vi "VisualizeNHRRGS.vi"() -> ()   [LabVIEW 2018, in "Visualization.lvlib" / "VisualizeAcPwr.lvclass"]
uses:
  VisualizeAcPwr.lvclass
  <vilib>/event_ctls.llb/usereventprio.ctl
  VisualizeBase/VisualizeBase_class/Requests/clUserEventType.ctl
  <vilib>/Utility/error.llb/Error Cluster From Error Code.vi
  <vilib>/ErrorRing/Error Ring.xnode
  VisualizeBase/VisualizeBase_class/VisualizeBase.lvclass
  <userlib>/NIST/NISTErrorLib/NISTErrorLib.lvlib
  AcPwr/AcPwrModule/AcPwrModule.lvlib
panel:
  out "Status Byte Register":T1(array[cluster])
  out "Incorrect DataType?":bool
  in  "PluginName":string="AcPwr.NHRRGS0"
  in  "PlotYAxis":u32[](array[numeric])=[0, 1, 0] max=1
  out "NHRRGS":waveform(dbl)[](graph)
  out "ErrorArray":errorcluster[](array[cluster])
  in  "QueuName":string="NHRRGSVQ"
  in  "btnStop":bool
  in  "btnReset":bool
  in  "btnClear":bool
  # "0=Left Axis and 1=Right Axis"
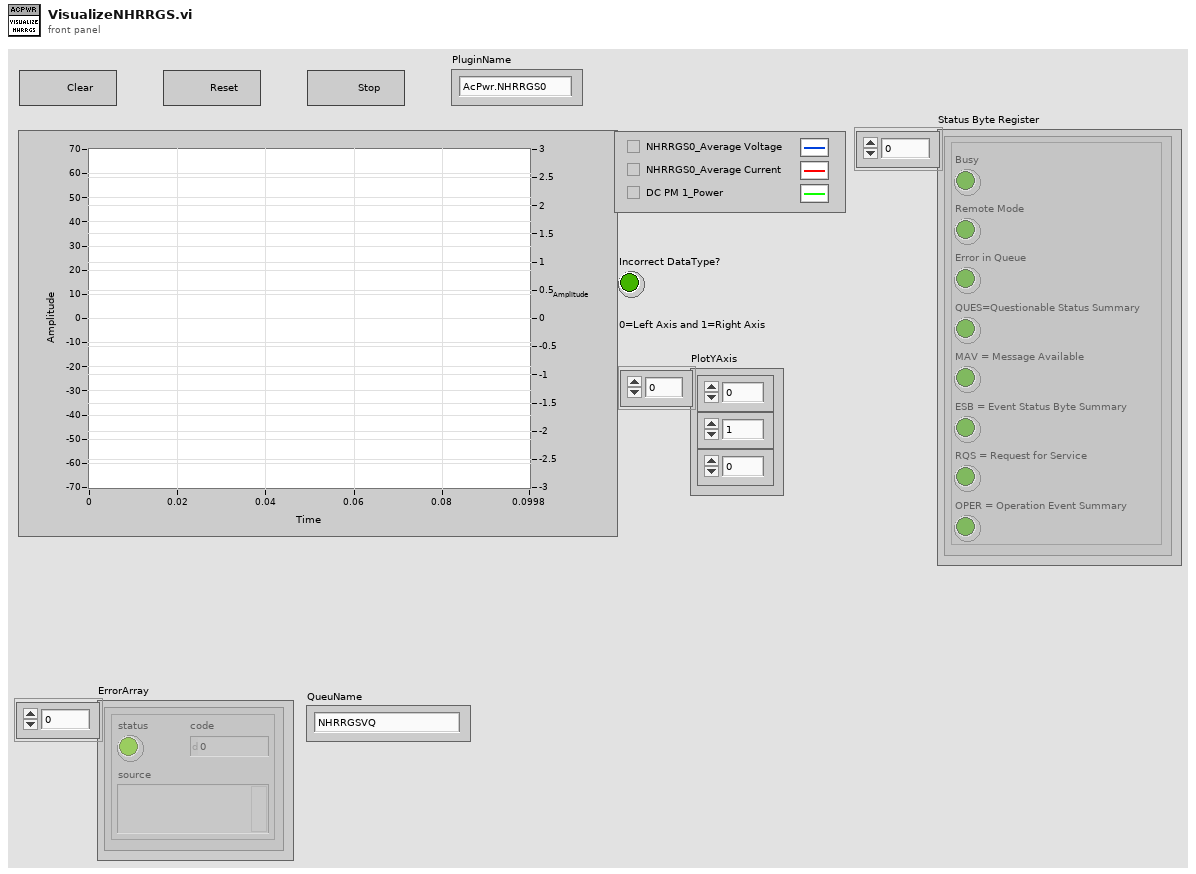
[diagram p1: front panel]
types:
  T1 = cluster{"Busy":bool, "Remote Mode":bool, "Error in Queue":bool, "QUES=Questionable Status Summary":bool, "MAV = Message Available":bool, "ESB = Event Status Byte Summary":bool, "RQS = Request for Service":bool, "OPER = Operation Event Summary":bool}[]
  T2 = typedef "Visualization.lvlib/VisualizeBase.lvclass/clRequestEvents.ctl" = cluster{"StopRequest":refnum<user-event>, "ResetRequest":refnum<user-event>}
  T3 = typedef "AcPwrModule.lvlib/clBroadcastEvents.ctl" = cluster{"DidInit":refnum<user-event>, "StatusUpdate":refnum<user-event>, "ErrorReport":refnum<user-event>, "DidStop":refnum<user-event>, "PathToINI":refnum<user-event>, "Measurements":refnum<user-event>, "LoadConfigFile":refnum<user-event>, "GetSettings":refnum<user-event>, "SetSettings":refnum<user-event>, "GetType&ID":refnum<user-event>, "GotSettings":refnum<user-event>}
  T4 = typedef "Visualization.lvlib/VisualizeBase.lvclass/clUserEventType.ctl" = cluster{"BusIndex":i8, "Data":variant}
  T5 = typedef "usereventprio.ctl" = enum32{"high priority", "normal priority"}
  T6 = cluster{"Busy":bool, "Remote Mode":bool, "Error in Queue":bool, "QUES = Questionable Status Summary":bool, "MAV = Message Available":bool, "ESB = Event Status Byte Summary":bool, "RQS = Request for Service":bool, "OPER = Operation Event Summary":bool}[]
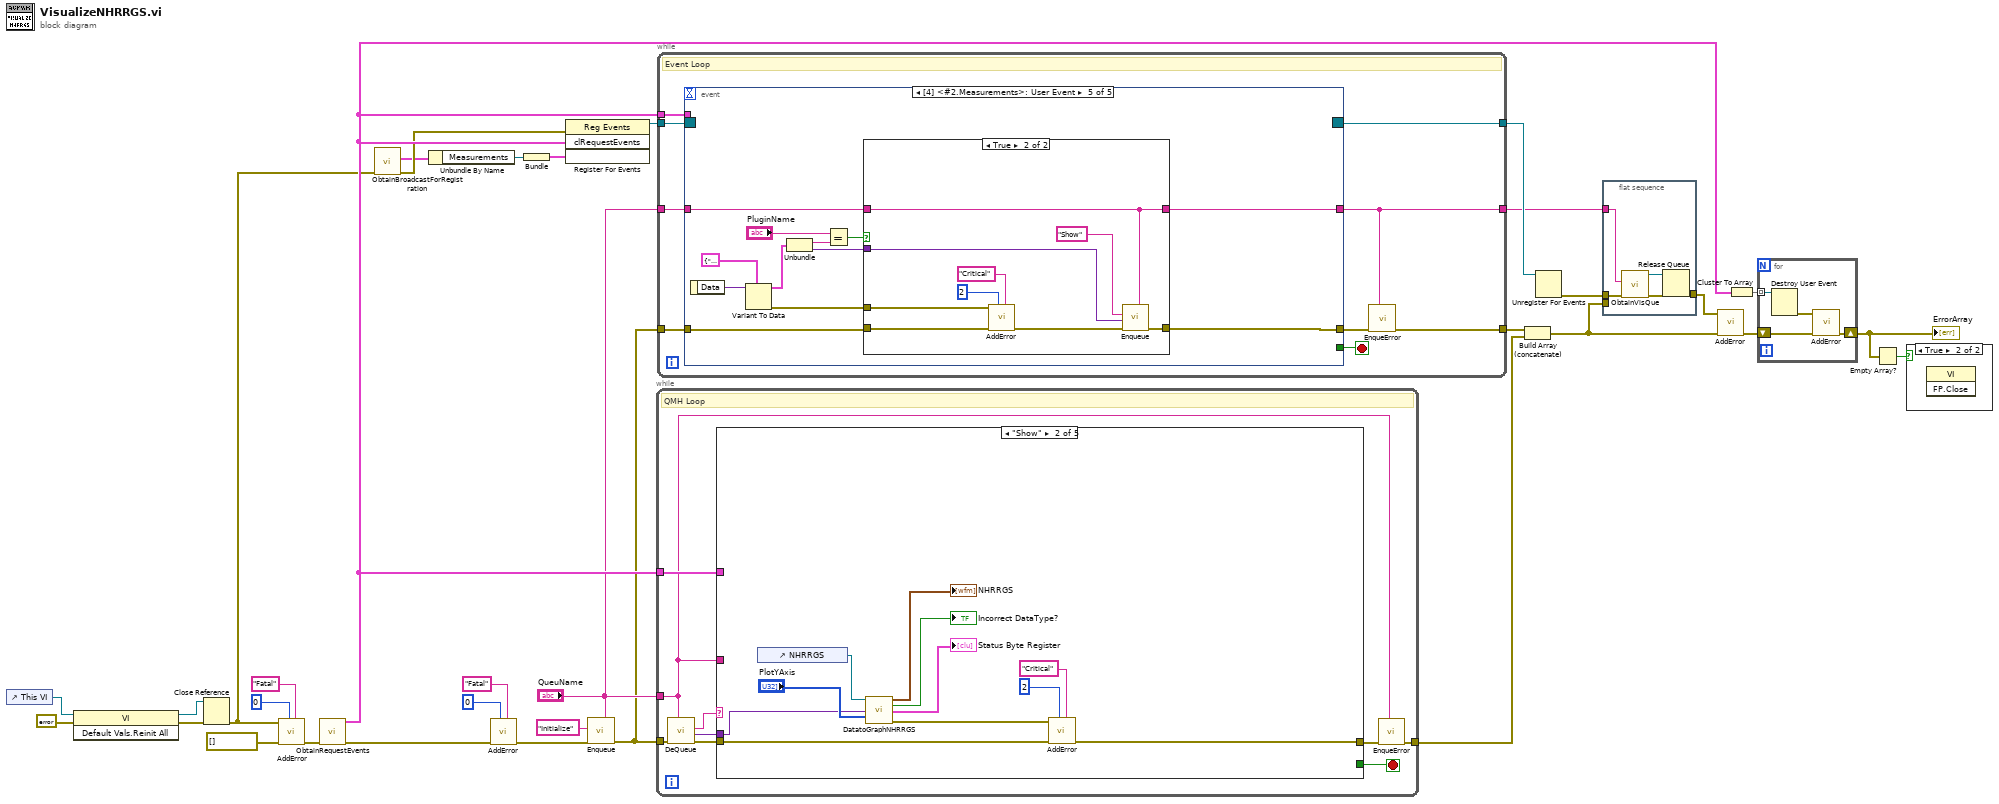
[diagram p0: block diagram]
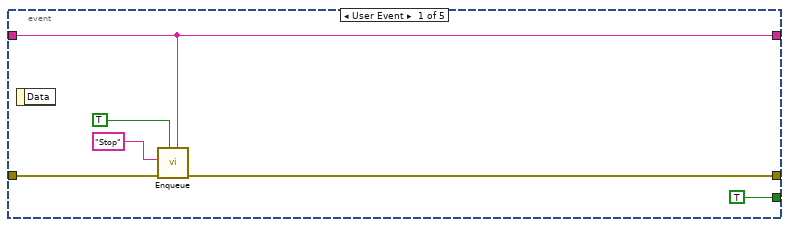
[diagram p2: hidden frame]
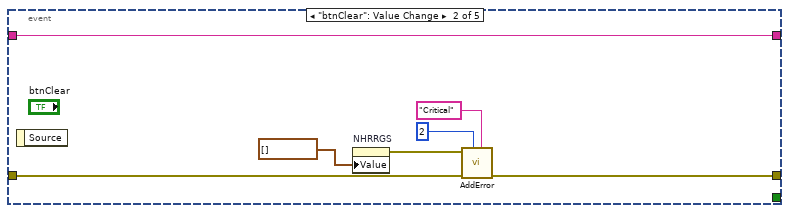
[diagram p3: hidden frame]
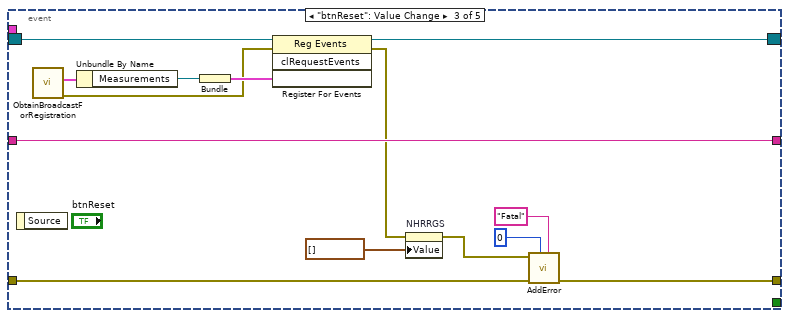
[diagram p4: hidden frame]
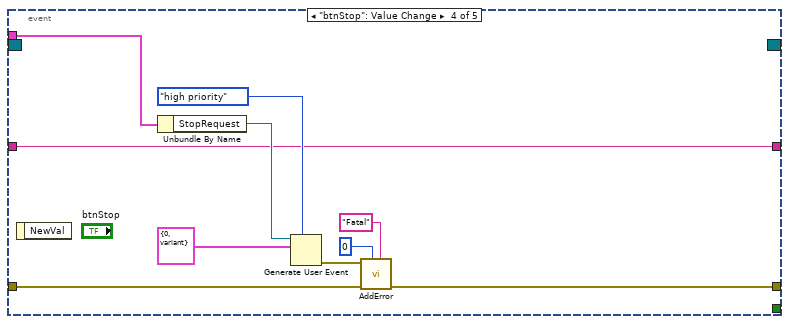
[diagram p5: hidden frame]
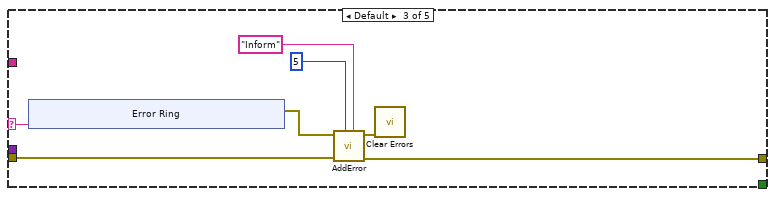
[diagram p8: hidden frame]
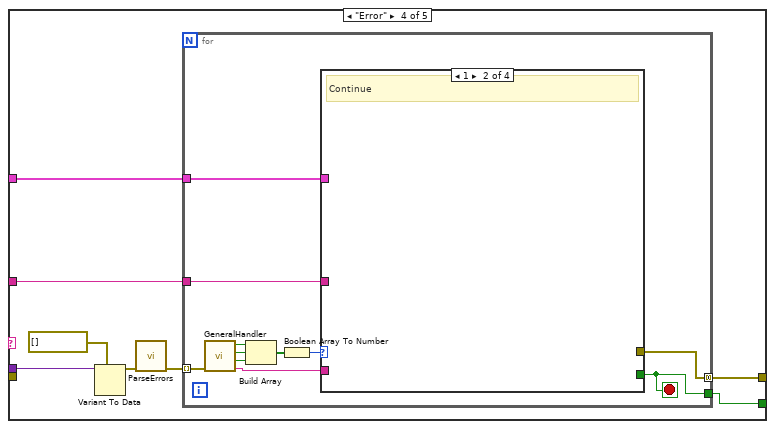
[diagram p9: hidden frame]
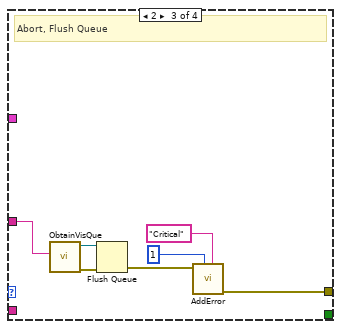
[diagram p11: hidden frame]
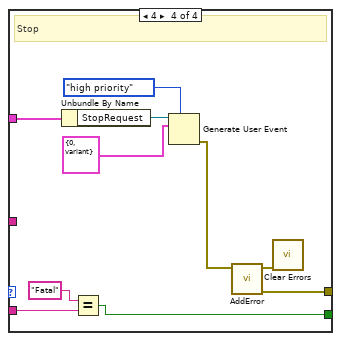
[diagram p12: hidden frame]
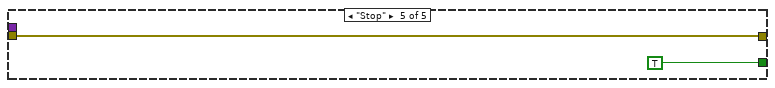
[diagram p13: hidden frame]
diagram:
  n1 = control-ref of="This VI"() -> (w19:refnum<vi>)
  n2 = invoke class="VI" method="Default Vals.Reinit All"(reference=w19, error in=errorcluster {"status"=FALSE, "code"=0, "source"=""} ("error in (no error)")) -> (reference out=w16:refnum<vi>, error out=w17:errorcluster)  [unwired: 1 in, 1 out]
  n3 = Close Reference(reference=w16, error in (no error)=w17) -> (error out=w14:errorcluster)
  n4 = call <userlib>:"AddError.vi"("Severity"="Fatal" ("String"), "Priority"=u8 0, "ErrorArray"=errorcluster[] [], "error in (no error)"=w14) -> ("ErrorArray"=w31:errorcluster[])  [unwired: 6 in, 1 out]
  n5 = call "ObtainRequestEvents.vi"("Error"=w31) -> ("Error"=w4:errorcluster[], "clRequestEvents"=w23:T2)  [unwired: 9 in]
  n6 = call "ObtainBroadcastForRegistration.vi"("error in (no error)"=w14) -> ("error out"=w13:errorcluster, "clBroadcastEvents"=w12:T3)  [unwired: 9 in]
  n7 = Unbundle By Name(w12) -> ("Measurements"=w21:refnum<user-event>)
  n8 = call <userlib>:"AddError.vi"("Severity"="Fatal" ("String"), "Priority"=u8 0, "ErrorArray"=w4) -> ("ErrorArray"=w3:errorcluster[])  [unwired: 7 in, 1 out]
  n9 = Bundle("Measurements"=w21) -> (w20:cluster{"Measurements":refnum<user-event>})  [unwired: 1 in]
  n10 = register-events(error in=w13, w23, w20) -> (reference out=w32:refnum<event-registration>)  [unwired: 1 in, 1 out]
  n11 = call "Enqueue.vi"("QueName"="QueuName", "Error"=w3, "Message"="Initialize") -> ("Error"=w2:errorcluster[])  [unwired: 8 in]
  n12 = while {
    tunnel: w2 -> [w42]
    tunnel: [w36] -> w27
    tunnel: "QueuName" -> [w34]
    tunnel: w23 -> [w35]
    stop <- w37 stop-if-true
    # "QMH Loop"
    n13 = call "DeQueue.vi"("QueName"=w34, "Error"=w42) -> ("Error"=w39:errorcluster[], "Data"=w40:variant, "Message"=w41:string)  [unwired: 7 in]
    n14 = case shown="\"Show\"" w41 {
      selector: w41 -> [_ _ w61 _ _]
      tunnel: w40 -> [_ w45 _ w76 _]
      tunnel: w39 -> [w43 w51 w59 _ w105]
      tunnel: [w43 w54 w58 w72 w105] -> w38
      tunnel: [_ _ _ w71 TRUE] -> w37
      tunnel: w35 -> [_ _ _ w70 _]
      tunnel: w34 -> [_ _ _ w69 _]
      frame "Initialize" {
      }
      frame "Show" {
        n15 = control-ref of="NHRRGS"() -> (w50:refnum<vi>)
        n16 = call "DatatoGraphNHRRGS.vi"("NHRRGS"=w50, "Data"=w45, "PlotYAxis"="PlotYAxis") -> ("WaveformArray"=→"NHRRGS":waveform(dbl)[], "Incorrect DataType?"=→"Incorrect DataType?":bool, "Status Byte Register"=→"Status Byte Register":T6, "error out"=w47:errorcluster)  [unwired: 9 in]
        n17 = call <userlib>:"AddError.vi"("Severity"="Critical" ("String"), "Priority"=u8 2, "ErrorArray"=w51, "error in (no error)"=w47) -> ("ErrorArray"=w54:errorcluster[])  [unwired: 6 in, 1 out]
      }
      frame Default {
        n18 = xnode "Error Ring"("parameter 0"=w61) -> ("error out"=w60:errorcluster)
        n19 = call <userlib>:"AddError.vi"("Severity"="Inform" ("String"), "Priority"=u8 5, "ErrorArray"=w59, "error in (no error)"=w60) -> ("ErrorArray"=w58:errorcluster[], "error out"=w57:errorcluster)  [unwired: 6 in]
        n20 = call <vilib>:"Clear Errors.vi"("error in (no error)"=w57) -> ()  [unwired: 5 in, 2 out]
      }
      frame "Error" {
        n21 = Variant To Data(type=errorcluster[] [], Variant=w76) -> (data=w74:errorcluster[])  [unwired: 1 in, 1 out]
        n22 = call <userlib>:"ParseErrors.vi"("ErrorArray"=w74) -> ("ErrorArray"=w73:errorcluster[])  [unwired: 8 in, 2 out]
        n23 = for {
          tunnel: w73 -> [w87] mode=indexing
          tunnel: [w81] -> w72 mode=concatenating
          tunnel: [w79] -> w71
          tunnel: w70 -> [w78]
          tunnel: w69 -> [w77]
          stop <- w79 stop-if-true
          n24 = call <userlib>:"GeneralHandler.vi"("error in (no error)"=w87) -> ("Severity"=w80:string, "Stop"=w84:bool, "Abort"=w85:bool, "Continue"=w86:bool)  [unwired: 7 in]
          n25 = Build Array(w86, w85, w84) -> (w83:bool[])
          n26 = Boolean Array To Number(Boolean array=w83) -> (number=w82:u32)
          n27 = case shown="1" w82 {
            tunnel: [_ _ w92 w103] -> w81
            tunnel: w80 -> [_ _ _ w98]
            tunnel: [_ _ _ w96] -> w79
            tunnel: w78 -> [_ _ _ w95]
            tunnel: w77 -> [_ _ w88 _]
            frame 0, Default {
              # "No Dialog"
            }
            frame 1 {
              # "Continue"
            }
            frame 2 {
              # "Abort, Flush Queue"
              n28 = call "ObtainVisQue.vi"("QueName"=w88) -> ("error out"=w94:errorcluster, "queue out"=w93:refnum<queue>)  [unwired: 9 in]
              n29 = Flush Queue(queue=w93, error in (no error)=w94) -> (error out=w91:errorcluster)  [unwired: 2 out]
              n30 = call <userlib>:"AddError.vi"("Severity"="Critical" ("String"), "Priority"=u8 1, "error in (no error)"=w91) -> ("ErrorArray"=w92:errorcluster[])  [unwired: 7 in, 1 out]
            }
            frame 4 {
              # "Stop"
              n31 = Unbundle By Name(w95) -> ("StopRequest"=w104:refnum<user-event>)
              n32 = Equal?(x="Fatal", y=w98) -> (x = y?=w96:bool)
              n33 = Generate User Event(priority (normal)=usereventprio."high priority", user event=w104, event data cluster=T4 {"BusIndex"=0, "Data"=variant} ("event data")) -> (error out=w102:errorcluster)  [unwired: 1 in, 1 out]
              n34 = call <userlib>:"AddError.vi"("error in (no error)"=w102) -> ("ErrorArray"=w103:errorcluster[], "error out"=w99:errorcluster)  [unwired: 9 in]
              n35 = call <vilib>:"Clear Errors.vi"("error in (no error)"=w99) -> ()  [unwired: 5 in, 2 out]
            }
          }
        }
      }
      frame "Stop" {
      }
    }
    n36 = call "EnqueError.vi"("QueName"=w34, "Error"=w38) -> ("Error"=w36:errorcluster[])  [unwired: 9 in]
  }
  n37 = while {
    tunnel: w32 -> [w115]
    tunnel: [w112] -> w28
    tunnel: [w111] -> w30
    tunnel: w23 -> [w110]
    tunnel: w2 -> [w109]
    tunnel: "QueuName" -> [w108]
    tunnel: [w107] -> w10
    stop <- w114 stop-if-true
    # "Event Loop"
    n38 = event shown="[4] <#2.Measurements>: User Event" {
      selector: w115 -> [_ _ w142 _ _]
      dyn-events: [_ _ w141 _ _] -> w111
      timeout: _ -> [_ _ _ _ _]
      tunnel: [TRUE _ _ _ _] -> w114
      tunnel: [w120 w125 w135 w150 w164] -> w113
      tunnel: w110 -> [_ _ _ w145 _]
      tunnel: w109 -> [w117 w124 w134 w143 w154]
      tunnel: w108 -> [w116 w128 w136 w144 w157]
      tunnel: [w116 w128 w136 w144 w156] -> w107
      event User Event {
        n39 = event-data() -> ()  [unwired: 1 in, 1 out]
        n40 = call "Enqueue.vi"("QueName"=w116, "Priority? (F)"=TRUE, "Error"=w117, "Message"="Stop") -> ("Error"=w120:errorcluster[])  [unwired: 7 in]
      }
      event "btnClear": Value Change {
        n41 = event-data() -> ()  [unwired: 1 in, 1 out]
        n42 = property on="NHRRGS" class="WFGraph (strict)"("Value"=waveform(dbl)[] [] ("NHRRGS")) -> (error out=w123:errorcluster)  [unwired: 2 in, 1 out]
        n43 = call <userlib>:"AddError.vi"("Severity"="Critical" ("String"), "Priority"=u8 2, "ErrorArray"=w124, "error in (no error)"=w123) -> ("ErrorArray"=w125:errorcluster[])  [unwired: 6 in, 1 out]
      }
      event "btnReset": Value Change {
        n44 = event-data() -> ()  [unwired: 1 in, 1 out]
        n45 = call "ObtainBroadcastForRegistration.vi"() -> ("error out"=w137:errorcluster, "clBroadcastEvents"=w138:T3)  [unwired: 10 in]
        n46 = Unbundle By Name(w138) -> ("Measurements"=w140:refnum<user-event>)
        n47 = Bundle("Measurements"=w140) -> (w139:cluster{"Measurements":refnum<user-event>})  [unwired: 1 in]
        n48 = register-events(reference=w142, error in=w137, w139) -> (reference out=w141:refnum<event-registration>, error out=w131:errorcluster)  [unwired: 1 in]
        n49 = property on="NHRRGS" class="WFGraph (strict)"(error in=w131, "Value"=waveform(dbl)[] [] ("NHRRGS")) -> (error out=w130:errorcluster)  [unwired: 1 in, 1 out]
        n50 = call <userlib>:"AddError.vi"("Severity"="Fatal" ("String"), "Priority"=u8 0, "ErrorArray"=w134, "error in (no error)"=w130) -> ("ErrorArray"=w135:errorcluster[])  [unwired: 6 in, 1 out]
      }
      event "btnStop": Value Change {
        n51 = event-data() -> ()  [unwired: 1 in, 1 out]
        n52 = Unbundle By Name(w145) -> ("StopRequest"=w151:refnum<user-event>)
        n53 = Generate User Event(priority (normal)=usereventprio."high priority", user event=w151, event data cluster=T4 {"BusIndex"=0, "Data"=variant} ("event data")) -> (error out=w152:errorcluster)  [unwired: 1 in, 1 out]
        n54 = call <userlib>:"AddError.vi"("Severity"="Fatal" ("String"), "Priority"=u8 0, "ErrorArray"=w143, "error in (no error)"=w152) -> ("ErrorArray"=w150:errorcluster[])  [unwired: 6 in, 1 out]
      }
      event User Event {
        n55 = event-data() -> ("Data"=w159:variant)  [unwired: 1 in]
        n56 = Variant To Data(type=cluster{string, "Data":variant} {"", "Data"=variant}, Variant=w159) -> (data=w162:cluster{string, "Data":variant}, error out=w153:errorcluster)  [unwired: 1 in]
        n57 = Unbundle(w162) -> (w161:string, "Data"=w155:variant)
        n58 = Equal?(x="PluginName", y=w161) -> (x = y?=w158:bool)
        n59 = case shown="True" w158 {
          tunnel: w155 -> [_ w175]
          tunnel: [w166 w173] -> w164
          tunnel: w154 -> [w166 w168]
          tunnel: w157 -> [w165 w172]
          tunnel: [w165 w172] -> w156
          tunnel: w153 -> [_ w167]
          frame False {
          }
          frame True {
            n60 = call <userlib>:"AddError.vi"("Severity"="Critical" ("String"), "Priority"=u8 2, "ErrorArray"=w168, "error in (no error)"=w167) -> ("ErrorArray"=w169:errorcluster[])  [unwired: 6 in, 1 out]
            n61 = call "Enqueue.vi"("QueName"=w172, "Error"=w169, "Data"=w175, "Message"="Show") -> ("Error"=w173:errorcluster[])  [unwired: 7 in]
          }
        }
      }
    }
    n62 = call "EnqueError.vi"("QueName"=w107, "Error"=w113) -> ("Error"=w112:errorcluster[])  [unwired: 9 in]
  }
  n63 = Build Array (concatenate)(w28, w27) -> (w1:errorcluster[])
  n64 = Unregister For Events(event registration refnum=w30) -> (error out=w26:errorcluster)  [unwired: 1 in]
  n65 = flat-sequence {
    tunnel: w26 -> [w180]
    tunnel: [w177] -> w25
    tunnel: w10 -> [w176]
    tunnel: w1 -> [_]
    frame #0 {
      n66 = call "ObtainVisQue.vi"("error in (no error)"=w180, "QueName"=w176) -> ("error out"=w179:errorcluster, "queue out"=w178:refnum<queue>)  [unwired: 8 in]
      n67 = Release Queue(queue=w178, error in (no error)=w179) -> (error out=w177:errorcluster)  [unwired: 1 in, 2 out]
    }
  }
  n68 = call <userlib>:"AddError.vi"("ErrorArray"=w1, "error in (no error)"=w25) -> ("ErrorArray"=w24:errorcluster[])  [unwired: 8 in, 1 out]
  n69 = Cluster To Array(cluster=w23) -> (array=w29:refnum<user-event>[])
  n70 = for {
    tunnel: w29 -> [w184] mode=indexing
    shift-right: [w183] -> w15
    shift-left: w24 -> [w182]
    n71 = Destroy User Event(user event=w184) -> (error out=w181:errorcluster)  [unwired: 1 in]
    n72 = call <userlib>:"AddError.vi"("ErrorArray"=w182, "error in (no error)"=w181) -> ("ErrorArray"=w183:errorcluster[])  [unwired: 8 in, 1 out]
  }
  "ErrorArray" <- w15
  n73 = Empty Array?(array=w15) -> (empty?=w22:bool)
  n74 = case shown="True" w22 {
    frame False {
    }
    frame True {
      n75 = invoke class="VI" method="FP.Close"() -> ()  [unwired: 3 in, 3 out]
    }
  }
